vi "threshold_cmp.vi"(0 "thresh_reset":bool, 5 "thresh_reset_index":u8, 9 "index":u8, 11 "value":fxp<+/-,32,16>) -> (2 "thresh_fault":bool, 4 "current_index":u8, 6 "current_minimum":fxp<+/-,32,16>, 8 "current_maximum":fxp<+/-,32,16>, 10 "current_ratio":u32, 15 "current_persistence":u32)   [LabVIEW 2018]
uses:
  <vilib>/rvi/Memory/Memory_Emulation/nirvimemoryFastEmulation.vi
  <vilib>/rvi/Memory/Memory_Emulation/nirvimemoryEmulation.vi
  <vilib>/rvi/Emulation/niFpgaEmulationIsFPGAContextNoSignature.vi
  <vilib>/rvi/DataTransferAndStorage/Container/Common/niFpgaContainerGetUniqueNameForEmu.vi
  <vilib>/rvi/Emulation/niFpgaProcessEmulError.vi
  <vilib>/rvi/Emulation/niFpgaSctlEmulationGetInTimedLoop.vi
  <vilib>/rvi/errors/nirviReportUnexpectedCaseInternalError (U32).vi
  <vilib>/rvi/DataTransferAndStorage/Container/XNode/niFpgaContainer.xnode
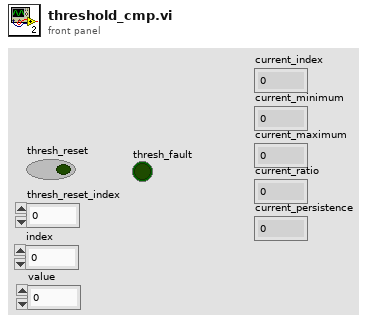
[diagram p1: front panel]
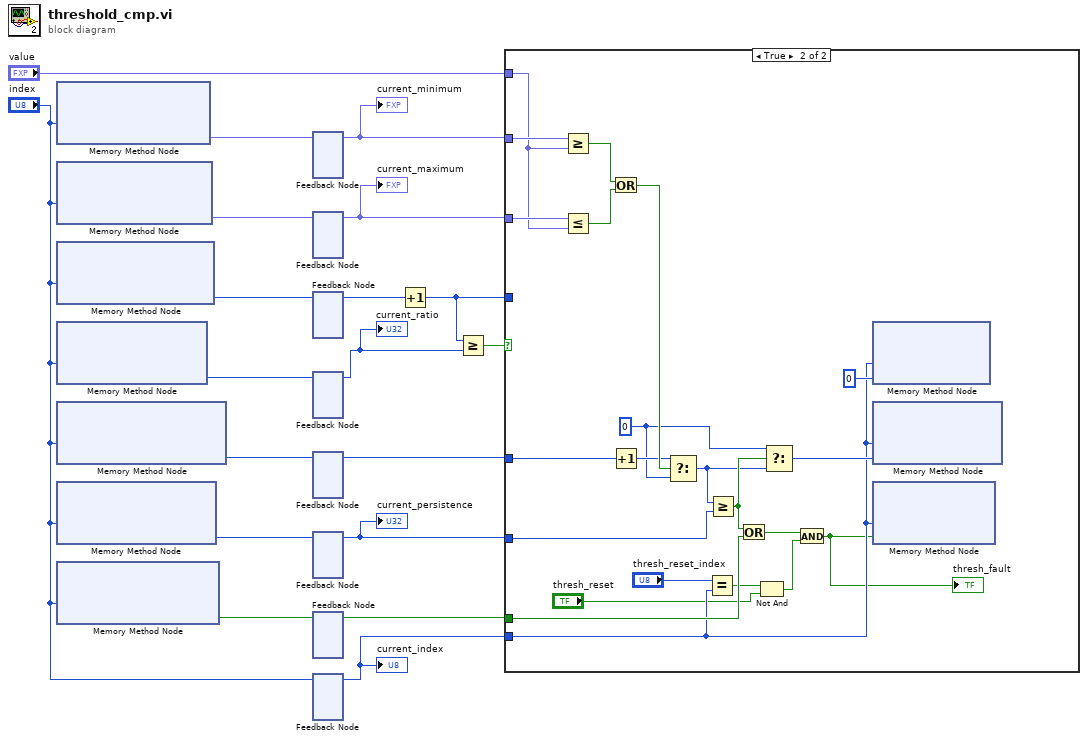
[diagram p0: block diagram]
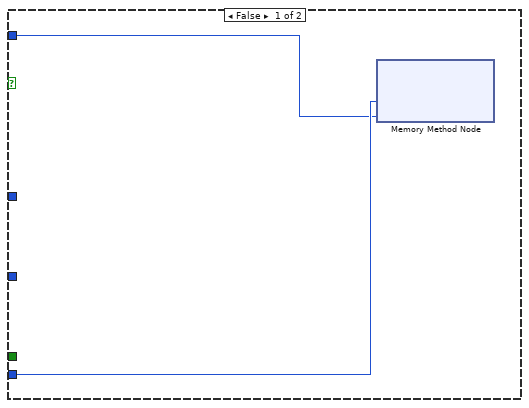
[diagram p2: hidden frame]
diagram:
  n1 = xnode ("Memory Method Node")("Address"="index") -> ("Data"=w4:fxp<+/-,32,16>)  [unwired: 1 in, 1 out]
  n2 = xnode ("Memory Method Node")("Address"="index") -> ("Data"=w6:fxp<+/-,32,16>)  [unwired: 1 in, 1 out]
  n3 = xnode ("Memory Method Node")("Address"="index") -> ("Data"=w9:u32)  [unwired: 1 in, 1 out]
  n4 = xnode ("Memory Method Node")("Address"="index") -> ("Data"=w10:u32)  [unwired: 1 in, 1 out]
  n5 = xnode ("Memory Method Node")("Address"="index") -> ("Data"=w14:u32)  [unwired: 1 in, 1 out]
  n6 = xnode ("Memory Method Node")("Address"="index") -> ("Data"=w13:u32)  [unwired: 1 in, 1 out]
  n7 = xnode ("Memory Method Node")("Address"="index") -> ("Data"=w12:bool)  [unwired: 1 in, 1 out]
  n8 = feedback #1() -> (w5:fxp<+/-,32,16>)  [unwired: 1 in]
  "current_minimum" <- w5
  n9 = feedback-in #1(w4) -> ()
  n10 = feedback #2() -> (w7:fxp<+/-,32,16>)  [unwired: 1 in]
  "current_maximum" <- w7
  n11 = feedback-in #2(w6) -> ()
  n12 = feedback #3() -> (w8:u32)  [unwired: 1 in]
  n13 = feedback-in #3(w9) -> ()
  n14 = feedback #4() -> (w11:u32)  [unwired: 1 in]
  "current_ratio" <- w11
  n15 = feedback-in #4(w10) -> ()
  n16 = feedback #5() -> (w15:u32)  [unwired: 1 in]
  n17 = feedback-in #5(w14) -> ()
  n18 = feedback #6() -> (w16:u32)  [unwired: 1 in]
  "current_persistence" <- w16
  n19 = feedback-in #6(w13) -> ()
  n20 = feedback #7() -> (w17:bool)  [unwired: 1 in]
  n21 = feedback-in #7(w12) -> ()
  n22 = feedback #8() -> (w18:u8)  [unwired: 1 in]
  "current_index" <- w18
  n23 = feedback-in #8("index") -> ()
  n24 = Increment(x=w8) -> (x+1=w3:u32)
  n25 = Greater Or Equal?(x=w3, y=w11) -> (x >= y?=w2:bool)
  n26 = case shown="True" w2 {
    tunnel: w5 -> [_ w43]
    tunnel: w7 -> [_ w42]
    tunnel: "value" -> [_ w41]
    tunnel: w15 -> [_ w37]
    tunnel: w16 -> [_ w35]
    tunnel: w17 -> [_ w34]
    tunnel: w18 -> [w21 w27]
    tunnel: w3 -> [w20 _]
    frame False {
      n27 = xnode ("Memory Method Node")("Address"=w21, "Data"=w20) -> ()  [unwired: 1 in, 1 out]
    }
    frame True {
      w29 = u32 0
      n28 = Greater Or Equal?(x=w43, y=w41) -> (x >= y?=w40:bool)
      n29 = Less Or Equal?(x=w42, y=w41) -> (x <= y?=w39:bool)
      n30 = Or(x=w40, y=w39) -> (x .or. y?=w38:bool)
      n31 = Increment(x=w37) -> (x+1=w36:u32)
      n32 = Select(t=w36, s=w38, f=w29) -> (s? t:f=w30:u32)
      n33 = Equal?(x="thresh_reset_index", y=w27) -> (x = y?=w24:bool)
      n34 = Greater Or Equal?(x=w30, y=w35) -> (x >= y?=w31:bool)
      n35 = Or(x=w31, y=w34) -> (x .or. y?=w33:bool)
      n36 = Not And(1:"thresh_reset", 2:w24) -> (0:w25:bool)
      n37 = Select(t=w29, s=w31, f=w30) -> (s? t:f=w28:u32)
      n38 = And(x=w33, y=w25) -> (x .and. y?=w22:bool)
      "thresh_fault" <- w22
      n39 = xnode ("Memory Method Node")("Address"=w27, "Data"=u32 0) -> ()  [unwired: 1 in, 1 out]
      n40 = xnode ("Memory Method Node")("Address"=w27, "Data"=w28) -> ()  [unwired: 1 in, 1 out]
      n41 = xnode ("Memory Method Node")("Address"=w27, "Data"=w22) -> ()  [unwired: 1 in, 1 out]
    }
  }
